vi "Remove Subscriptions by Index.vi"(8 "error in (no error)":errorcluster, 10 "Index of Elements to Remove":i32[](array[numeric]), 11 "MVC Subscription in":refnum<class "MVC Subscription.lvclass">) -> (0 "error out":errorcluster, 3 "MVC Subscription out":refnum<class "MVC Subscription.lvclass">)   [LabVIEW 2016, in "MVC Subscription.lvlib" / "MVC Subscription.lvclass"]
uses:
  MVC Subscription.lvclass
  MVC Subscription.lvclass/MVC Subscription.ctl
  <userlib>/_OpenG.lib/array/array.llb/Delete Elements from 1D Array (Variant)__ogtk.vi
  <vilib>/ActorFramework/Message Enqueuer/Message Enqueuer.lvclass
  <vilib>/ActorFramework/Message/Message.lvclass
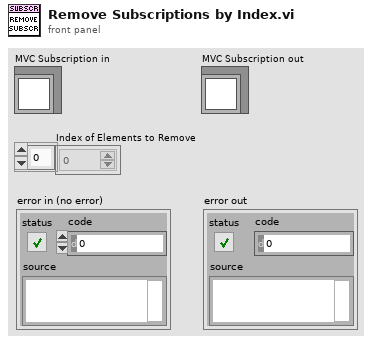
[diagram p1: front panel]
types:
  T1 = typedef "MVC Subscription.lvlib/MVC Subscription.lvclass/Cluster - Individual Subscription.ctl" = cluster{"Enqueuer":refnum<class "Message Enqueuer.lvclass">, "Message":refnum<class "Message.lvclass">}
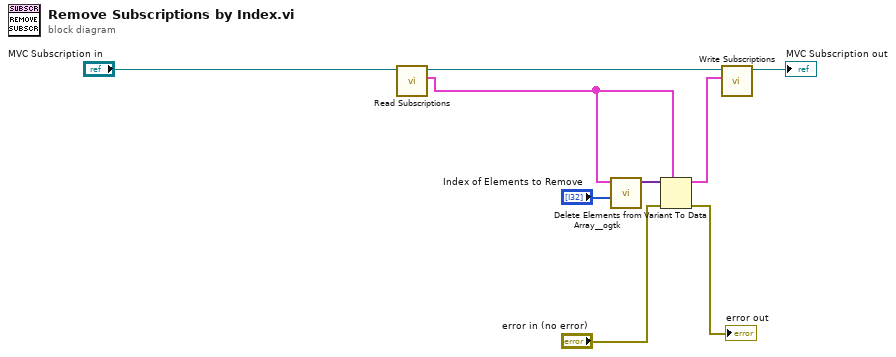
[diagram p0: block diagram]
diagram:
  n1 = call "Read Subscriptions.vi"("MVC Subscription in"="MVC Subscription in") -> ("Subscriptions"=w8:T1[], "MVC Subscription out"=w7:refnum<class "MVC Subscription.lvclass">)  [unwired: 9 in]
  n2 = call-poly <userlib>:"Delete Elements from Array__ogtk.vi"("indices"="Index of Elements to Remove", "array"=w8) -> ("array w/ subset deleted"=w3:variant[])  [unwired: 8 in, 1 out]
  n3 = Variant To Data(error in="error in (no error)", type=w8, Variant=w3) -> (data=w5:T1[], error out=→"error out":errorcluster)
  n4 = call "Write Subscriptions.vi"("Subscriptions"=w5, "MVC Subscription in"=w7) -> ("MVC Subscription out"=→"MVC Subscription out":refnum<class "MVC Subscription.lvclass">)  [unwired: 9 in]
